vi "init_COM_inter.vi"(0 "VISA Refnum in":refnum<visa-resource-name>) -> (14 "VISA out":refnum<visa-resource-name>, 15 "HTTP client handle out":T1, 17 "Internet OK":bool, 19 "VISA error out":errorcluster)   [LabVIEW 2016]
uses:
  <vilib>/httpClient/ClientHandle.ctl
  <vilib>/Utility/error.llb/DialogType.ctl
  <vilib>/Instr/_visa.llb/VISA Configure Serial Port (Instr).vi
  <vilib>/httpClient/LabVIEWHTTPClient.lvlib
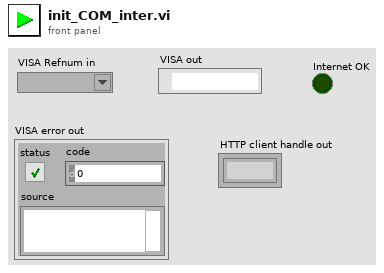
[diagram p1: front panel]
types:
  T1 = typedef "LabVIEWHTTPClient.lvlib/ClientHandle.ctl" = refnum<k1>
  T2 = typedef "DialogType.ctl" = u16
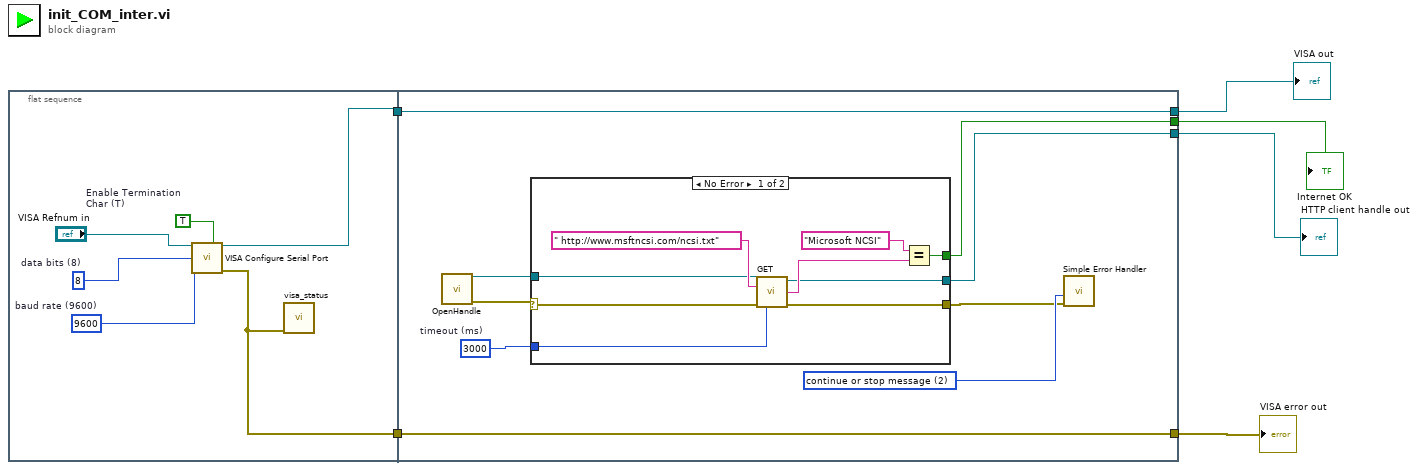
[diagram p0: block diagram]
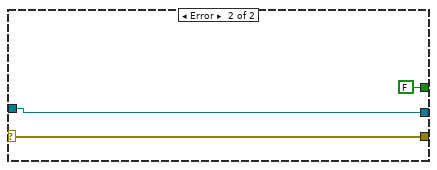
[diagram p2: hidden frame]
diagram:
  n1 = flat-sequence {
    tunnel: [w8] -> w6
    tunnel: [w7] -> w4
    tunnel: w6 -> [w16]
    tunnel: w4 -> [w15]
    tunnel: [w16] -> w5
    tunnel: [w15] -> w3
    tunnel: [w14] -> w2
    tunnel: [w13] -> w1
    frame #0 {
      w9 = u16 8  # data bits (8)
      w10 = TRUE  # Enable Termination Char (T)
      w11 = u32 9600  # baud rate (9600)
      n2 = call-poly "VISA Configure Serial Port"("VISA resource name"="VISA Refnum in", "Enable Termination\nChar (T)"=w10, "baud rate (9600)"=w11, "data bits (8)"=w9) -> ("VISA resource name out"=w8:refnum<visa-resource-name>, "error out"=w7:errorcluster)  [unwired: 10 in]
      n3 = call "visa_status.vi"("error in (no error)"=w7) -> ()  [unwired: 11 in]
    }
    frame #1 {
      w18 = T2 2 items=["no dialog", "OK message", "continue or stop message", "OK message + warnings", "continue/stop + warnings"] ("type of dialog (OK msg:1)")
      w21 = 3000  # timeout (ms)
      n4 = call <vilib>:"OpenHandle.vi"() -> ("client handle out"=w19:T1, "error out"=w20:errorcluster)  [unwired: 14 in]
      n5 = case shown="No Error" w20 {
        selector: w20 -> [w25 w32]
        tunnel: [w27 FALSE] -> w14
        tunnel: [w26 w32] -> w17
        tunnel: w21 -> [w24 _]
        tunnel: w19 -> [w23 w31]
        tunnel: [w22 w31] -> w13
        frame No Error {
          n6 = call <vilib>:"GET.vi"("client handle"=w23, "url"=" http://www.msftncsi.com/ncsi.txt" ("address"), "error in (no error)"=w25, "timeout (10000)"=w24) -> ("client handle out"=w22:T1, "body"=w28:string, "error out"=w26:errorcluster)  [unwired: 8 in, 1 out]
          n7 = Equal?(x="Microsoft NCSI", y=w28) -> (x = y?=w27:bool)
        }
        frame Error {
        }
      }
      n8 = call <vilib>:"Simple Error Handler.vi"("type of dialog (OK msg:1)"=w18, "error in (no error)"=w17) -> ()  [unwired: 3 in, 5 out]
    }
  }
  "VISA out" <- w5
  "VISA error out" <- w3
  "Internet OK" <- w2
  "HTTP client handle out" <- w1
